vi "ble_cmd_system_reset.vi"(8 "error in (no error)":errorcluster, 11 "COM Bluegiga in":refnum<visa-resource-name>) -> (0 "error out":errorcluster, 3 "COM Bluegiga out":refnum<visa-resource-name>)   [LabVIEW 2017]
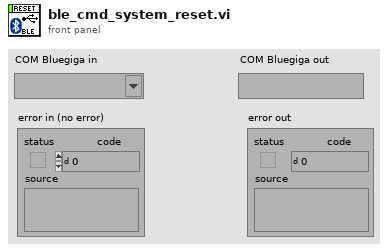
[diagram p1: front panel]
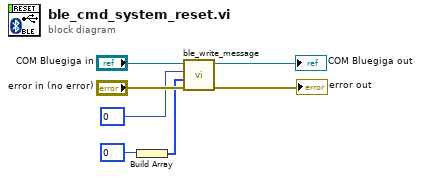
[diagram p0: block diagram]
diagram:
  n1 = Build Array(u8 0 ("Message ID (0x00)")) -> (w3:u8[])
  n2 = call "ble_write_message.vi"("error in (no error)"="error in (no error)", "Payload(Empty)"=w3, "Message ID (0x00)"=u8 0, "COM Bluegiga in"="COM Bluegiga in") -> ("error out"=→"error out":errorcluster, "COM Bluegiga out"=→"COM Bluegiga out":refnum<visa-resource-name>)  [unwired: 5 in, 1 out]
